vi "SDSU_DacRegsAliases.vi"(10 "cmd in":string) -> (0 "alias converted":bool, 1 "register?":bool, 2 "cmds out":string[](array[string]), 3 "first reg":i32)   [LabVIEW 2016]
panel:
  out "Array":string[](array[string])
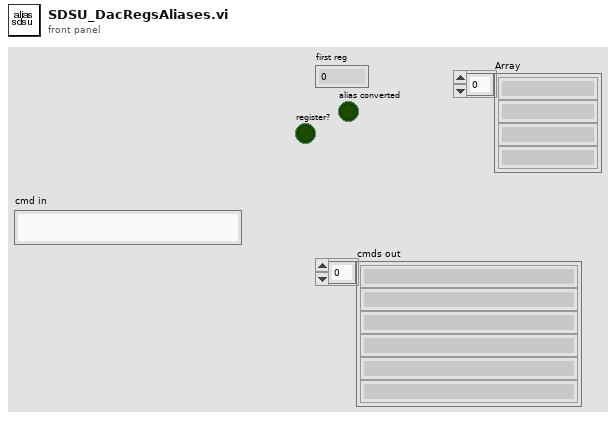
[diagram p1: front panel]
types:
  T1 = enum16{"read from file", "find", "get", "add", "delete", "clear "}
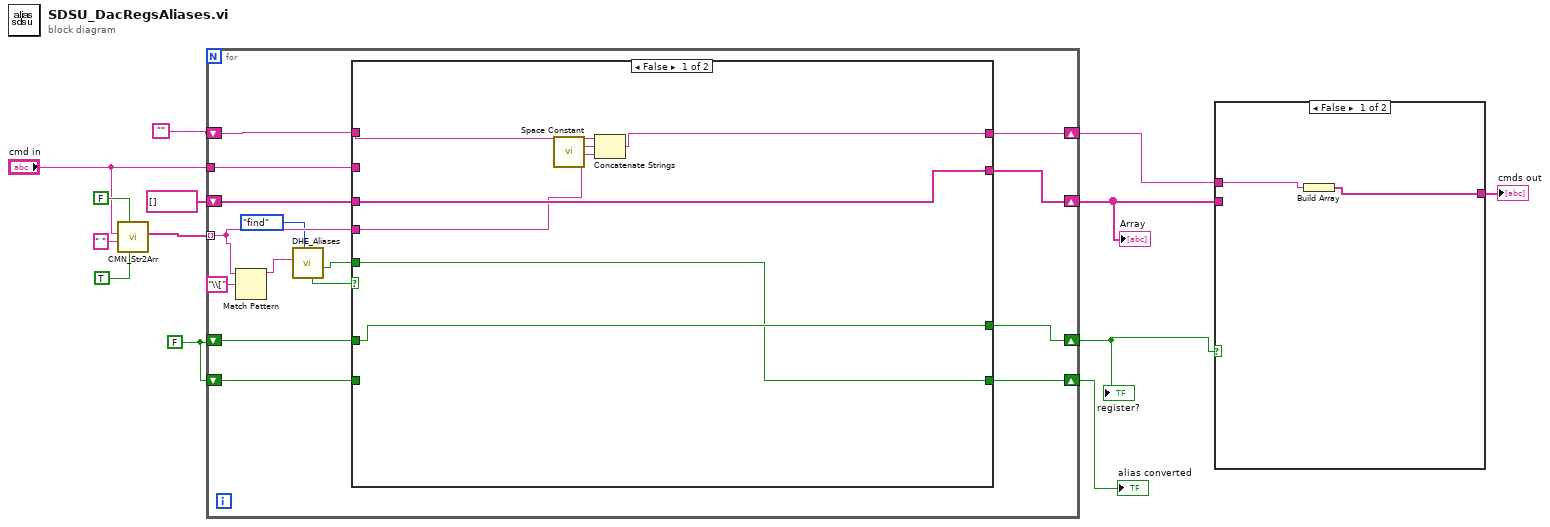
[diagram p0: block diagram]
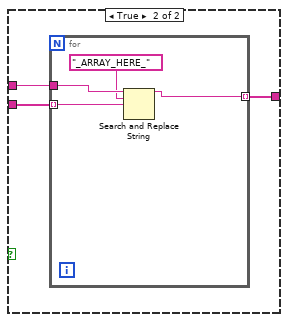
[diagram p2: hidden frame]
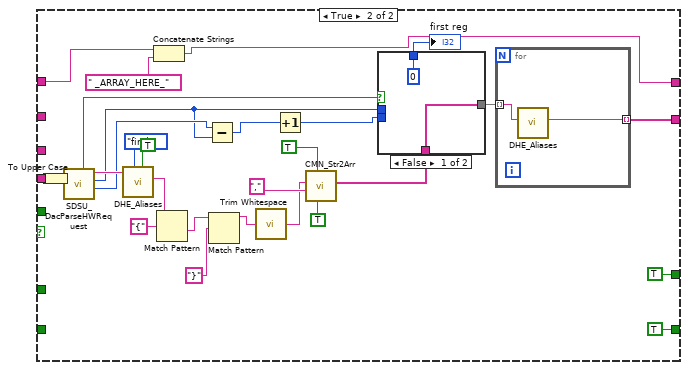
[diagram p3: hidden frame]
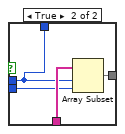
[diagram p4: hidden frame]
diagram:
  w3 = FALSE
  n1 = call "CMN_Str2Arr.vi"("trim"=TRUE, "strip quotation marks"=FALSE, "separator"=" ", "string in"="cmd in") -> ("Array out"=w10:string[])  [unwired: 7 in]
  n2 = for {
    tunnel: w10 -> [w25] mode=indexing
    shift-right: [w23] -> w6
    shift-left: "" -> [w24]
    shift-right: [w21] -> w7
    shift-left: w3 -> [w22]
    shift-right: [w20] -> w4
    shift-left: string[] [] -> [w19]
    shift-right: [w16] -> w2
    shift-left: w3 -> [w15]
    tunnel: "cmd in" -> [w14]
    n3 = Match Pattern(string=w25, regular expression="\\[") -> (before substring=w26:string)  [unwired: 1 in, 3 out]
    n4 = call "DHE_Aliases.vi"("action"=T1."find", "name in"=w26) -> ("found?"=w18:bool, "register?"=w28:bool)  [unwired: 6 in, 2 out]
    n5 = case shown="False" w28 {
      tunnel: w25 -> [w31 w63]
      tunnel: w24 -> [w35 w43]
      tunnel: [w34 w41] -> w23
      tunnel: w22 -> [w33 _]
      tunnel: [w33 TRUE] -> w21
      tunnel: [w32 w39] -> w20
      tunnel: w19 -> [w32 _]
      tunnel: w18 -> [w30 _]
      tunnel: [w30 TRUE] -> w16
      tunnel: w15 -> [_ _]
      tunnel: w14 -> [_ _]
      frame False {
        n6 = call <vilib>:"Space Constant.vi"() -> ("String"=w29:string)
        n7 = Concatenate Strings(w35, w29, w31) -> (w34:string)
      }
      frame True {
        n8 = To Upper Case(1:w63) -> (0:w38:string)
        n9 = call "SDSU_DacParseHWRequest.vi"("requested value"=w38) -> ("last reg"=w50:i32, "first reg"=w49:i32, "name out"=w62:string, "partial?"=w44:bool)  [unwired: 6 in, 1 out]
        n10 = call "DHE_Aliases.vi"("expand reg"=TRUE, "action"=T1."find", "name in"=w62) -> ("name out"=w58:string)  [unwired: 5 in, 3 out]
        n11 = Concatenate Strings(w43, " _ARRAY_HERE_" ("string")) -> (w41:string)
        n12 = Match Pattern(string=w58, regular expression="{") -> (after substring=w56:string)  [unwired: 1 in, 3 out]
        n13 = Subtract(x=w50, y=w49) -> (x-y=w48:i32)
        n14 = Match Pattern(string=w56, regular expression="}") -> (before substring=w46:string)  [unwired: 1 in, 3 out]
        n15 = call <vilib>:"Trim Whitespace.vi"("string"=w46) -> ("trimmed string"=w54:string)  [unwired: 1 in]
        n16 = Increment(x=w48) -> (x+1=w45:i32)
        n17 = call "CMN_Str2Arr.vi"("trim"=TRUE, "strip quotation marks"=TRUE, "separator"=",", "string in"=w54) -> ("Array out"=w51:string[])  [unwired: 7 in]
        n18 = case shown="False" w44 {
          tunnel: w51 -> [w65 w69]
          tunnel: w49 -> [_ w66]
          tunnel: [w65 w68] -> w47
          tunnel: w45 -> [_ w67]
          tunnel: [0 ("first reg") w66] -> w37
          frame False {
          }
          frame True {
            n19 = Array Subset(array=w69, index=w66, length=w67) -> (w68:string[])
          }
        }
        "first reg" <- w37
        n20 = for {
          tunnel: w47 -> [w71] mode=indexing
          tunnel: [w70] -> w39 mode=indexing
          n21 = call "DHE_Aliases.vi"("name in"=w71) -> ("name out"=w70:string)  [unwired: 7 in, 3 out]
        }
      }
    }
  }
  "register?" <- w7
  "Array" <- w4
  "alias converted" <- w2
  n22 = case shown="False" w7 {
    tunnel: w4 -> [_ w76]
    tunnel: w6 -> [w73 w75]
    tunnel: [w72 w74] -> w5
    frame False {
      n23 = Build Array(w73) -> (w72:string[])
    }
    frame True {
      n24 = for {
        tunnel: w76 -> [w78] mode=indexing
        tunnel: w75 -> [w80]
        tunnel: [w77] -> w74 mode=indexing
        n25 = Search and Replace String(input string=w80, search string="_ARRAY_HERE_" ("string"), replace string=w78) -> (result string=w77:string)  [unwired: 5 in, 3 out]
      }
    }
  }
  "cmds out" <- w5
